vi "uManagerWriteTXT.vi"(4 "numImg":u32, 5 "expTime":dbl, 6 "error in (no error)":errorcluster, 7 "start":dbl, 8 "file path labViewCom":path, 9 "file path AcqSettings":path) -> (0 "error out":errorcluster)   [LabVIEW 2021]
panel:
  out "AcqSettingsOut":string
  out "labViewComOut":string
  out "labViewCom":string="Start: 1; ExpTime: 10; NumOfImages: 100;"
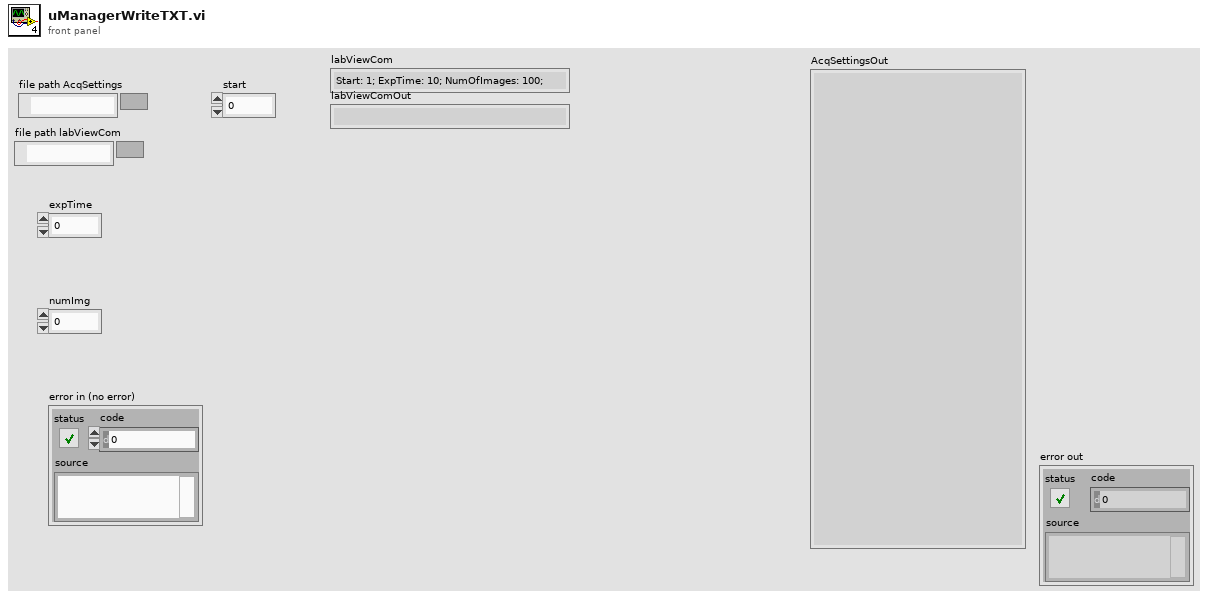
[diagram p1: front panel]
types:
  T1 = enum16{"open", "replace", "create", "open or create", "replace or create", "replace or create with confirmation"}
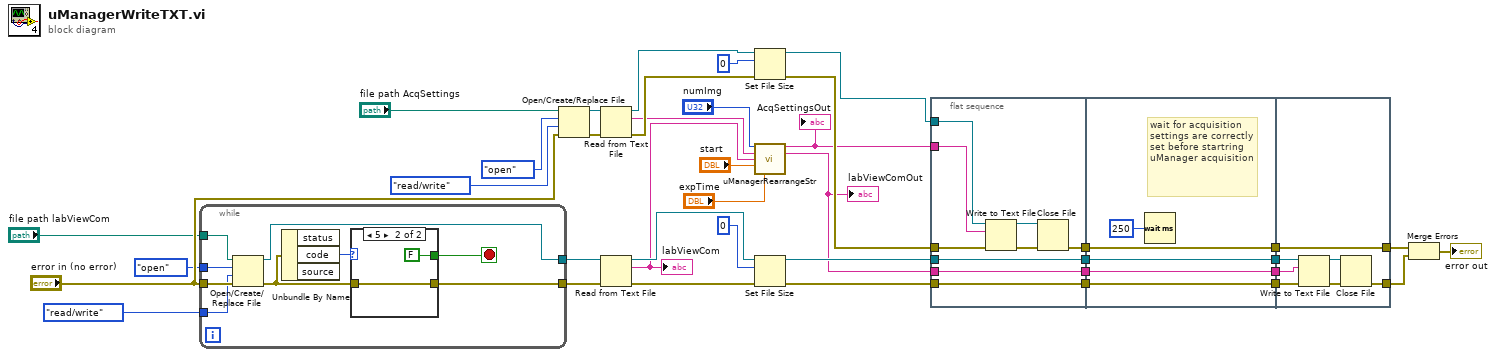
[diagram p0: block diagram]
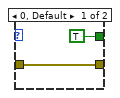
[diagram p2: hidden frame]
diagram:
  n1 = while {
    tunnel: "error in (no error)" -> [w48]
    tunnel: [w47] -> w17
    tunnel: enum16{"read/write", "read-only", "write-only"}."read/write" ("access (0:read/write)") -> [w46]
    tunnel: T1."open" ("operation (0:open)") -> [w45]
    tunnel: "file path labViewCom" -> [w44]
    tunnel: [w40] -> w1
    stop <- w41 stop-if-true
    n2 = Open/Create/Replace File(file path (use dialog)=w44, error in=w48, operation (0:open)=w45, access (0:read/write)=w46) -> (refnum out=w47:refnum<file>, error out=w42:errorcluster)  [unwired: 2 in, 1 out]
    n3 = Unbundle By Name(w42) -> ("code"=w43:i32)  [unwired: 2 out]
    n4 = case shown="5" w43 {
      tunnel: [TRUE FALSE] -> w41
      tunnel: w42 -> [w49 w51]
      tunnel: [w49 w51] -> w40
      frame 0, Default {
      }
      frame 5 {
      }
    }
  }
  n5 = Open/Create/Replace File(file path (use dialog)="file path AcqSettings", error in="error in (no error)", operation (0:open)=T1."open", access (0:read/write)=enum16{"read/write", "read-only", "write-only"}."read/write") -> (refnum out=w22:refnum<file>, error out=w23:errorcluster)  [unwired: 2 in, 1 out]
  n6 = Read from Text File(file (use dialog)=w22, error in=w23) -> (refnum out=w35:refnum<file>, text=w29:string, error out=w38:errorcluster)  [unwired: 2 in, 1 out]
  n7 = Read from Text File(file (use dialog)=w17, error in=w1) -> (refnum out=w31:refnum<file>, text=w25:string, error out=w30:errorcluster)  [unwired: 2 in, 1 out]
  "labViewCom" <- w25
  n8 = Set File Size(4:w38, 6:i64 0 ("size (in bytes)"), 7:w35) -> (0:w39:errorcluster, 3:w36:refnum<file>)
  n9 = call "uManagerRearrangeStr.vi"("numImg"="numImg", "AcqSettingsIn"=w29, "labViewComIn"=w25, "start"="start", "expTime"="expTime") -> ("AcqSettingsOut"=w33:string, "labViewComOut"=w8:string)  [unwired: 9 in]
  "labViewComOut" <- w8
  "AcqSettingsOut" <- w33
  n10 = Set File Size(4:w30, 6:i64 0 ("offset (in bytes) (0)"), 7:w31) -> (0:w5:errorcluster, 3:w11:refnum<file>)
  n11 = flat-sequence {
    tunnel: w39 -> [w61]
    tunnel: w36 -> [w60]
    tunnel: w33 -> [w59]
    tunnel: [w54] -> w13
    tunnel: w11 -> [w58]
    tunnel: [w58] -> w10
    tunnel: w8 -> [w57]
    tunnel: [w57] -> w6
    tunnel: w5 -> [w56]
    tunnel: [w56] -> w3
    tunnel: w13 -> [w66]
    tunnel: [w66] -> w12
    tunnel: w10 -> [w65]
    tunnel: [w65] -> w9
    tunnel: [w64] -> w7
    tunnel: w6 -> [w64]
    tunnel: [w63] -> w4
    tunnel: w3 -> [w63]
    tunnel: [w73] -> w34
    tunnel: w12 -> [w73]
    tunnel: w9 -> [w72]
    tunnel: w7 -> [w71]
    tunnel: w4 -> [w70]
    tunnel: [w67] -> w2
    frame #0 {
      n12 = Write to Text File(file (use dialog)=w60, text=w59, error in=w61) -> (refnum out=w53:refnum<file>, error out=w55:errorcluster)  [unwired: 1 in, 1 out]
      n13 = Close File(refnum=w53, error in=w55) -> (error out=w54:errorcluster)  [unwired: 1 out]
    }
    frame #1 {
      # "wait for acquisition settings are correctly set before startring uManager acquisition"
      n14 = Wait (ms)(milliseconds to wait=u32 250) -> ()  [unwired: 1 out]
    }
    frame #2 {
      n15 = Write to Text File(file (use dialog)=w72, text=w71, error in=w70) -> (refnum out=w69:refnum<file>, error out=w68:errorcluster)  [unwired: 1 in, 1 out]
      n16 = Close File(refnum=w69, error in=w68) -> (error out=w67:errorcluster)  [unwired: 1 out]
    }
  }
  n17 = Merge Errors(w34, w2) -> (→"error out":errorcluster)
